vi "WS1050_VSA_AD7747 Updated.vi"(0 "Select Com S0":refnum<visa-resource-name>="COM1", 1 "Voltage P1":refnum<visa-resource-name>="GPIB0::9::INSTR", 2 "OFFSet Cal":dbl, 3 "Data Record Path":path=path "S:/ProductDevelopmentProjects/Work/ProductTest/Package Test/QL3B/QL3BW19_HTOL_A_T0HRS/Self_Actuation_Data_10_Parts", 4 "Voltage File Path":path=path "S:/Software_Control/RELEASED_SOFTWARE_RUN_ALL_TEST_FROM_HERE/PACKAGE/TMN/CS-TEST-SYSTEM/VSA_Voltage_Seq_0-35 to 43-43 to 35-0V.txt", 5 "OFFSet Cal 2":dbl, 6 "OFFSet Cal 3":dbl, 7 "error in (no error)":errorcluster, 8 "Header Table":string[][](table)=[["Lot#", "Wafer#", "SN#", "Stress Test", "Test_Run", "Temp", "Op", "Result", "I_Dvdd", "I_total", "I_vdd1"], ["QL1", "8", "3", "3X-HTOL", "96Hrs", "25", "HG", "FAIL", "74.85E-6", "74.83E-6", ""]], 11 "input cluster":T1) -> (12 "VSA_V3":string, 13 "C1_Max(pF)_V1":string, 14 "VSA_V1":string, 15 "C2_Max(pF)_V1":string, 16 "Voltage P1 Out":refnum<visa-resource-name>, 17 "C3_Max(pF)_V3":string, 18 "VSA_V 2":string, 19 "Com Out":refnum<visa-resource-name>, 20 "Status":string, 21 "C3_Max(pF)_V1":string, 22 "C1_Max_V2 (pF)":string, 23 "C1_Max(pF)_V3":string, 24 "C2_Max(pF)_V3":string, 25 "C2_Max_V2 (pF)":string, 26 "C3_Max_V2 (pF)":string, 27 "error out":errorcluster)   [LabVIEW 2017]
uses:
  Andy's LLB LV2012/Read_Test_Limits/TSTR Configuration Cluster1.0.ctl
panel:
  out "V_Out":dbl=30.0
  in  "o/pHeader Table":string[][](table)
  # "TMN CS Self Actuation Test System Ver1.2"
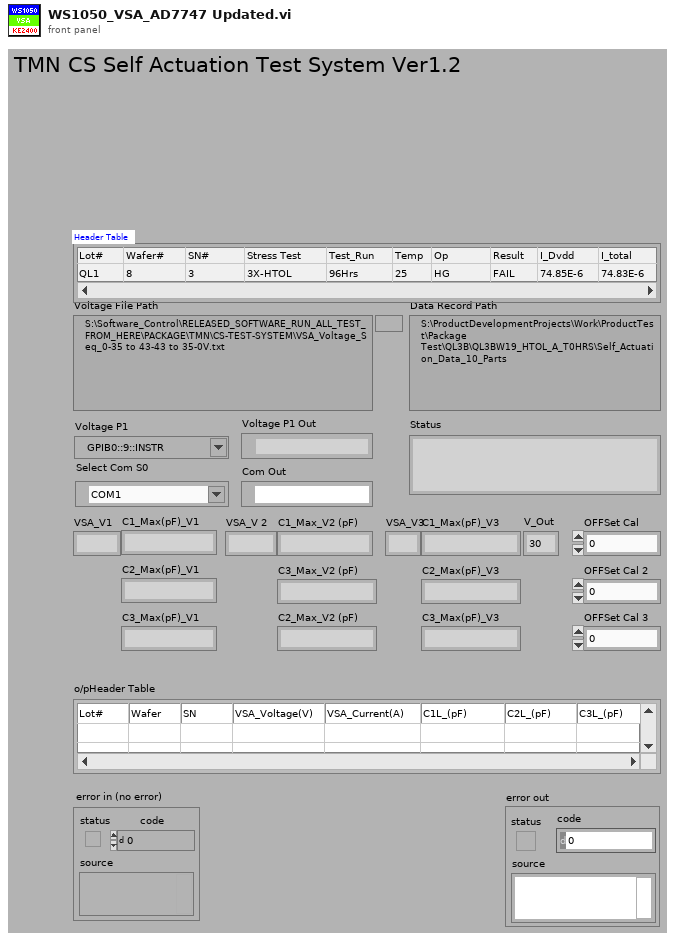
[diagram p1: front panel]
types:
  T1 = typedef "TSTR Configuration Cluster1.0.ctl" = cluster{"DeltaCA Low Limit ":dbl, "DeltaCA High Limit (V)":dbl, "DeltaCE Low Limit ":dbl, "DeltaCE High Limit":dbl, "DeltaCC Low Limit":dbl, "DeltaCC High Limit":dbl, "RTZ Limit":dbl, "Cmin Low Limit":dbl, "Cmin High Limit":dbl, "Idd High Limit (A)":dbl, "Idd Low Limit (A)":dbl, "Delta IDD":dbl, "Bin Path":string, "VSA Path1":string, "Dem Path":string, "Delay":dbl, "VSA":bool, "SWCyc":bool, "VPI":bool, "Bipolar":bool, "OVS Voltage":dbl, "Wait Time":dbl, "ATE":bool, "VNA GPIB":string, "Meter GPIB ":string, "Op level":string, "Idd Standby":dbl, "VSA Voltage1":dbl, "VSA Cap":dbl, "Test Name":string, "Nominal Trim Code":i32, "VPI Trim Code":i32, "De-Embd":bool, "Loop Count":i32, "Bipolar":bool, "VSA Path 2":string, "VSA Voltage2":dbl}
  T2 = enum16{"open", "replace", "create", "open or create", "replace or create", "replace or create with confirmation"}
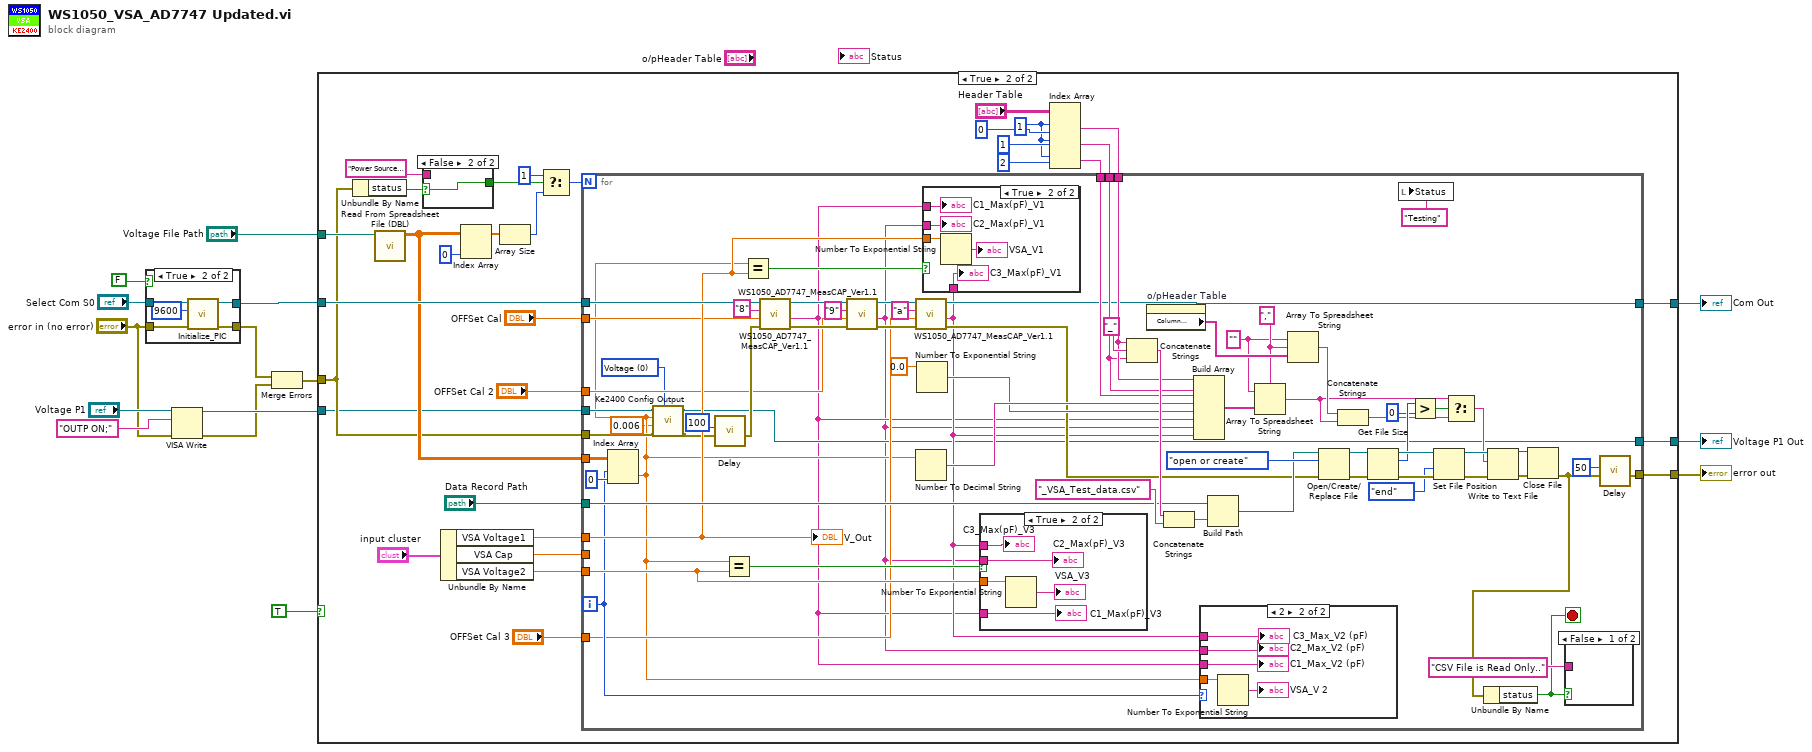
[diagram p0: block diagram]
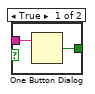
[diagram p4: hidden frame]
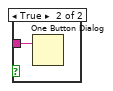
[diagram p8: hidden frame]
diagram:
  n1 = case shown="True" FALSE {
    tunnel: [w16 w22] -> w3
    tunnel: [w17 w21] -> w13
    tunnel: "Select Com S0" -> [w17 w20]
    tunnel: "error in (no error)" -> [w16 w19]
    frame False {
    }
    frame True {
      n2 = call "Initialize_PIC.vi"("error in (no error)"=w19, "baud rate"=u32 9600, "Select Com Port"=w20) -> ("error out"=w22:errorcluster, "VISA resource name out"=w21:refnum<visa-resource-name>)  [unwired: 7 in]
    }
  }
  n3 = VISA Write(VISA resource name="Voltage P1", write buffer="OUTP ON;", error in (no error)="error in (no error)") -> (VISA resource name out=w5:refnum<visa-resource-name>, error out=w2:errorcluster)  [unwired: 1 out]
  n4 = Merge Errors(w3, w2) -> (w1:errorcluster)
  n5 = case shown="True" TRUE {
    tunnel: w5 -> [w24 w26]
    tunnel: w1 -> [w25 w27]
    tunnel: [w24 w33] -> w9
    tunnel: [w25 w34] -> w10
    tunnel: w13 -> [w23 w38]
    tunnel: [w23 w32] -> w11
    tunnel: "Voltage File Path" -> [_ w28]
    frame False {
    }
    frame True {
      w46 = 1 ("disabled index (col)")
      n6 = Unbundle By Name(w27) -> ("status"=w39:bool)
      n7 = call <vilib>:"Read From Spreadsheet File (DBL).vi"("file path (dialog if empty)"=w28) -> ("all rows"=w37:dbl[][])  [unwired: 3 in, 7 out]
      n8 = case shown="False" w39 {
        selector: w39 -> [_ w60]
        tunnel: [w59 w60] -> w52
        tunnel: "Power Source \nNot Connected" ("Status") -> [w58 _]
        frame True {
          n9 = One Button Dialog(message=w58) -> (true=w59:bool)  [unwired: 1 out]
        }
        frame False {
        }
      }
      n10 = Unbundle By Name("input cluster") -> ("VSA Voltage1"=w40:dbl, "VSA Cap"=w41:dbl, "VSA Voltage2"=w35:dbl)
      n11 = Index Array(array=w37, index (col)=0 ("disabled index (col)")) -> (element=w57:dbl[])  [unwired: 1 in]
      n12 = Array Size(array=w57) -> (size(s)=w53:i32)
      n13 = Select(t=1 ("disabled index (col)"), s=w52, f=w53) -> (s? t:f=w36:i32)
      n14 = Index Array(array="Header Table", index (row) #1=w46, index (col) #1=0 ("disabled index (col)"), index (row) #2=w46, index (col) #2=1 ("disabled index (col)"), index (row) #3=w46, index (col) #3=2 ("disabled index (col)")) -> (element #1=w45:string, element #2=w44:string, element #3=w43:string)
      n15 = for {
        N: w36 -> [_]
        tunnel: w37 -> [w131]
        tunnel: w26 -> [w71]
        tunnel: "Data Record Path" -> [w95]
        tunnel: w27 -> [w73]
        tunnel: [w70] -> w33
        tunnel: [w64] -> w34
        tunnel: w45 -> [w98]
        tunnel: w44 -> [w97]
        tunnel: w43 -> [w96]
        tunnel: w41 -> [_]
        tunnel: w40 -> [w83]
        tunnel: w38 -> [w101]
        tunnel: w35 -> [w84]
        tunnel: [w79] -> w32
        tunnel: "OFFSet Cal" -> [w76]
        tunnel: "OFFSet Cal 2" -> [w75]
        tunnel: "OFFSet Cal 3" -> [w74]
        i -> [w78]
        stop <- w102 stop-if-true
        w67 = u16 0 items=["Voltage", "Current"] ("Source Mode  (0: Voltage)")
        w108 = "," ("delimiter (Tab)")
        w107 = "" ("format string")
        n16 = Index Array(array=w131, index (row)=w78, index (col)=0 ("disabled index (col)")) -> (element=w69:dbl)
        n17 = call "Ke2400 Config Output.vi"("Source Mode  (0: Voltage)"=w67, "error in (no error)"=w73, "Compliance  Level (0.1)"=0.006, "Output Level (0)"=w69, "VISA resource name"=w71) -> ("error out"=w72:errorcluster, "VISA resource name out"=w70:refnum<visa-resource-name>)  [unwired: 5 in]
        n18 = call "Delay.vi"("error in (no error)"=w72, "milliseconds to wait"=u32 100) -> ("error out"=w91:errorcluster)  [unwired: 9 in]
        n19 = Equal?(x=w69, y=w84) -> (x = y?=w85:bool)
        n20 = Equal?(x=w69, y=w83) -> (x = y?=w86:bool)
        n21 = call "WS1050_AD7747_MeasCAP_Ver1.1.vi"("error in (no error)"=w91, "OFFSet Cal"=w76, "AD7747_Number"="8", "Control"=w101) -> ("error"=w94:errorcluster, "CAP (pF)"=w66:string, "Control out"=w93:refnum<visa-resource-name>)  [unwired: 3 in, 2 out]
        n22 = call "WS1050_AD7747_MeasCAP_Ver1.1.vi"("error in (no error)"=w94, "OFFSet Cal"=w75, "AD7747_Number"="9", "Control"=w93) -> ("error"=w82:errorcluster, "CAP (pF)"=w65:string, "Control out"=w80:refnum<visa-resource-name>)  [unwired: 3 in, 2 out]
        n23 = call "WS1050_AD7747_MeasCAP_Ver1.1.vi"("error in (no error)"=w82, "OFFSet Cal"=w74, "AD7747_Number"="a", "Control"=w80) -> ("error"=w81:errorcluster, "CAP (pF)"=w77:string, "Control out"=w79:refnum<visa-resource-name>)  [unwired: 3 in, 2 out]
        n24 = Number To Decimal String(number=w69) -> (decimal integer string=w90:string)  [unwired: 1 out]
        n25 = Number To Exponential String(number=0.0) -> (E-format string=w89:string)  [unwired: 3 out]
        n26 = case shown="True" w86 {
          tunnel: w83 -> [_ w146]
          tunnel: w66 -> [_ w144]
          tunnel: w65 -> [_ w143]
          tunnel: w77 -> [_ w142]
          frame False {
          }
          frame True {
            n27 = Number To Exponential String(number=w146) -> (E-format string=→"VSA_V1":string)  [unwired: 3 out]
            "C2_Max(pF)_V1" <- w143
            "C1_Max(pF)_V1" <- w144
            "C3_Max(pF)_V1" <- w142
          }
        }
        n28 = case shown="True" w85 {
          tunnel: w84 -> [_ w141]
          tunnel: w77 -> [_ w139]
          tunnel: w66 -> [_ w138]
          tunnel: w65 -> [_ w137]
          frame False {
          }
          frame True {
            n29 = Number To Exponential String(number=w141) -> (E-format string=→"VSA_V3":string)  [unwired: 3 out]
            "C3_Max(pF)_V3" <- w139
            "C1_Max(pF)_V3" <- w138
            "C2_Max(pF)_V3" <- w137
          }
        }
        n30 = Concatenate Strings(w98, "_" ("format string"), w97) -> (w99:string)
        n31 = property on="o/pHeader Table" class="Tbl (strict)"() -> ("Column Headers[]"=w110:string[])  [unwired: 2 in, 2 out]
        n32 = Concatenate Strings(w99, "_VSA_Test_data.csv" ("name or relative path")) -> (w111:string)
        n33 = Build Array(w98, w97, w96, w90, w89, w66, w65, w77) -> (w109:string[])
        n34 = case shown="2" w78 {
          tunnel: w69 -> [_ w135]
          tunnel: w77 -> [_ w134]
          tunnel: w65 -> [_ w133]
          tunnel: w66 -> [_ w132]
          frame 0, Default {
          }
          frame 2 {
            n35 = Number To Exponential String(number=w135) -> (E-format string=→"VSA_V 2":string)  [unwired: 3 out]
            "C3_Max_V2 (pF)" <- w134
            "C2_Max_V2 (pF)" <- w133
            "C1_Max_V2 (pF)" <- w132
          }
        }
        n36 = Build Path(base path=w95, name or relative path=w111) -> (appended path=w122:path)
        n37 = Array To Spreadsheet String(delimiter (Tab)=w108, array=w109, 3:w107) -> (spreadsheet string=w106:string)
        n38 = Array To Spreadsheet String(delimiter (Tab)=w108, array=w110, 3:w107) -> (spreadsheet string=w118:string)
        n39 = Open/Create/Replace File(file path (use dialog)=w122, error in=w81, operation (0:open)=T2."open or create") -> (refnum out=w130:refnum<file>, error out=w125:errorcluster)  [unwired: 4 out]
        n40 = Concatenate Strings(w118, w106) -> (w117:string)
        n41 = Get File Size(file=w130, error in=w125) -> (refnum out=w129:refnum<file>, size (in bytes)=w121:i64, 0:w127:errorcluster)
        n42 = local write "Status"("Testing" ("Status")) -> ()
        n43 = Greater?(x=w121, y=i64 0) -> (0:w119:bool)
        n44 = Set File Position(refnum=w129, from (0:start)=enum16{"start", "end", "current"}."end", error in=w127) -> (refnum out=w128:refnum<file>, error out=w126:errorcluster)  [unwired: 1 out]
        n45 = Select(t=w106, s=w119, f=w117) -> (s? t:f=w116:string)
        n46 = Write to Text File(file (use dialog)=w128, text=w116, error in=w126) -> (refnum out=w114:refnum<file>, error out=w115:errorcluster)  [unwired: 2 out]
        n47 = Close File(refnum=w114, error in=w115) -> (error out=w63:errorcluster)  [unwired: 1 out]
        n48 = Unbundle By Name(w63) -> ("status"=w102:bool)
        n49 = case shown="False" w102 {
          tunnel: "CSV File is Read Only.." ("delimiter (Tab)") -> [_ w147]
          frame False {
          }
          frame True {
            n50 = One Button Dialog(message=w147) -> ()  [unwired: 2 out]
          }
        }
        n51 = call "Delay.vi"("error in (no error)"=w63, "milliseconds to wait"=u32 50) -> ("error out"=w64:errorcluster)  [unwired: 9 in]
        "V_Out" <- w83
      }
    }
  }
  "Voltage P1 Out" <- w9
  "Com Out" <- w11
  "error out" <- w10
